vi "Guessing Game.vi"() -> ()   [LabVIEW 2012]
doc: "This VI is an exercise in the LabVIEW Core I course.\n\nEnter the number of columns and rows you want generated, then run the VI. This VI generates an array with the number of rows and columns you specify."
panel:
  out "Waveform Chart":dbl(graph)
  in  "Min in":dbl
  in  "Max in":dbl
  out "Error Message":string
  out "Guess":dbl
  out "# of Guesses":i32
  in  "Min":dbl format="%#.6f"
  in  "Max":dbl=10000000.0 format="%#.6f"
  in  "Your Number":dbl format="%#.6f"
  # "Choose a range (i.e. Max and Min)\nThen choose \"Your Number\" that is \nin that range. Then run code."
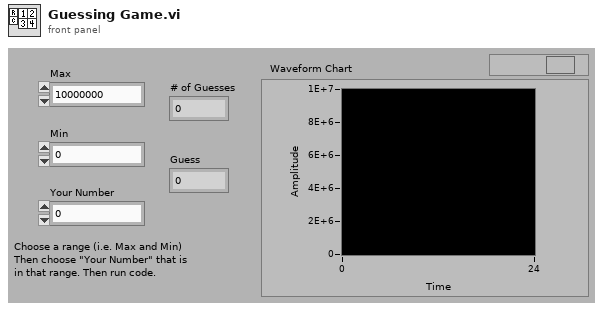
[diagram p1: front panel]
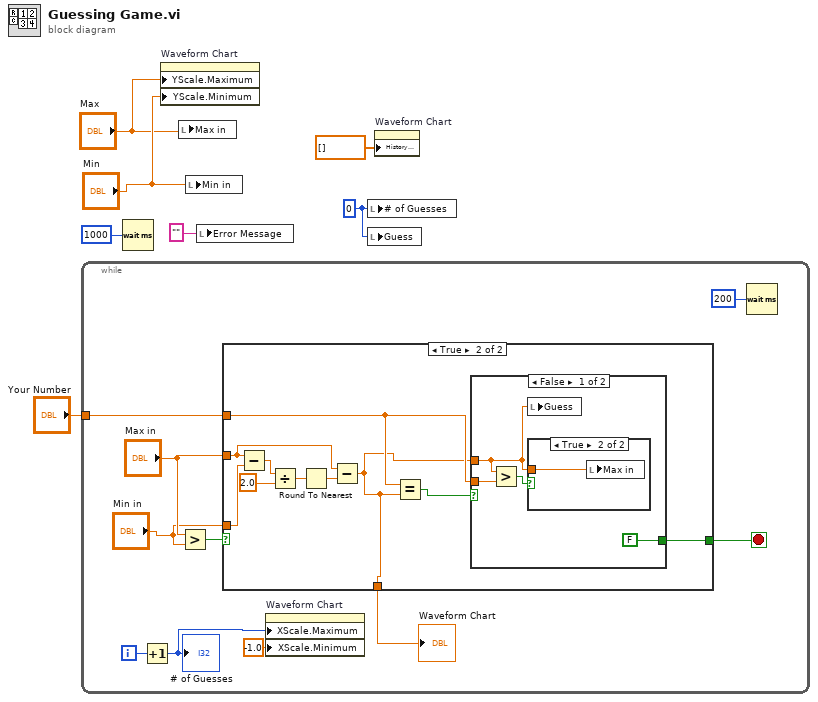
[diagram p0: block diagram]
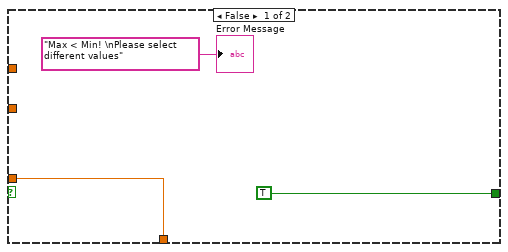
[diagram p2: hidden frame]
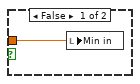
[diagram p3: hidden frame]
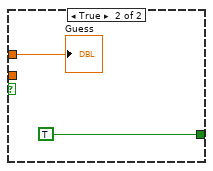
[diagram p4: hidden frame]
diagram:
  w7 = 0 ("# of Guesses")
  n1 = while {
    tunnel: "Your Number" -> [w13]
    i -> [w17]
    stop <- w14 stop-if-true
    n2 = Increment(x=w17) -> (x+1=w8:i32)
    "# of Guesses" <- w8
    n3 = Greater?(x="Max in", y="Min in") -> (0:w16:bool)
    n4 = case shown="True" w16 {
      tunnel: [TRUE w27] -> w14
      tunnel: w13 -> [_ w23]
      tunnel: "Min in" -> [w18 w29]
      tunnel: "Max in" -> [_ w25]
      tunnel: [w18 w21] -> w10
      frame False {
        "Error Message" <- "Max < Min! \nPlease select different values" ("Error Message")
      }
      frame True {
        n5 = Subtract(x=w25, y=w29) -> (x-y=w28:dbl)
        n6 = Divide(x=w28, y=2.0) -> (x/y=w26:dbl)
        n7 = Round To Nearest(number=w26) -> (nearest integer value=w24:dbl)
        n8 = Subtract(x=w25, y=w24) -> (x-y=w21:dbl)
        n9 = Equal?(x=w23, y=w21) -> (x = y?=w22:bool)
        n10 = case shown="False" w22 {
          tunnel: w21 -> [w31 w38]
          tunnel: w23 -> [w34 _]
          tunnel: [FALSE TRUE] -> w27
          frame False {
            n11 = Greater?(x=w31, y=w34) -> (0:w33:bool)
            n12 = local write "Guess"(w31) -> ()
            n13 = case shown="True" w33 {
              tunnel: w31 -> [w35 w36]
              frame False {
                n14 = local write "Min in"(w35) -> ()
              }
              frame True {
                n15 = local write "Max in"(w36) -> ()
              }
            }
          }
          frame True {
            "Guess" <- w38
          }
        }
      }
    }
    "Waveform Chart" <- w10
    n16 = property on="Waveform Chart" class="WFChart (strict)"("XScale.Maximum"=w8, "XScale.Minimum"=-1.0 ("Y Scale.Range:Minimum")) -> ()  [unwired: 2 in, 2 out]
    n17 = Wait (ms)(milliseconds to wait=u32 200) -> ()  [unwired: 1 out]
  }
  n18 = Wait (ms)(milliseconds to wait=u32 1000) -> ()  [unwired: 1 out]
  n19 = property on="Waveform Chart" class="WFChart (strict)"("YScale.Maximum"="Max", "YScale.Minimum"="Min") -> ()  [unwired: 2 in, 2 out]
  n20 = local write "Max in"("Max") -> ()
  n21 = local write "Min in"("Min") -> ()
  n22 = local write "Error Message"("" ("Error Message")) -> ()
  n23 = local write "# of Guesses"(w7) -> ()
  n24 = local write "Guess"(w7) -> ()
  n25 = property on="Waveform Chart" class="WFChart (strict)"("History Data"=dbl[] []) -> ()  [unwired: 2 in, 2 out]
